vi "RunMe.vi"() -> ()   [LabVIEW 2011]
uses:
  Documenti/Globals.vi
  <vilib>/gmath/NI_Gmath.lvlib
panel:
  in  "Sensor side":enum16{"Right", "Left"}(ring)
  out "Position":dbl(knob) max=500.0 scale=0.0..360.0
  out "home?":bool=TRUE
  in  "Motor on":bool
  out "Measurement OK":bool
  in  "stop":bool
  in  "Tab Control":enum32{"Connect", "Acquire", "Analyze"}(tab)
  in  "Sphere tolerance (mm)":dbl=0.5
  in  "Sphere nominal diameter (mm)":dbl=12.5
  in  "VISA resource name":refnum<visa-resource-name>
  out "pulses":u32
  out "Progress Bar":u32(slide) max=500 scale=-1.0..500.0
  in  "Record Button":bool
  out "data":enum16{"Right", "Left"}(ring)
  out "Current measurement":cluster{dbl[], dbl[]}(graph)
  out "Previus measurements":cluster{dbl[], "best nonlinear fit":dbl[]}[](graph)
  in  "index (page)":i32=1 min=-1 step=1
  out "Residuals":cluster{dbl[], dbl[]}(graph)
  in  "model description":T1={"model"="r+n*sin(x/360*2*3.141593+f)", "Parameters"=["r", "n", "f"], "x"="x"}
  in  "initial parameters":dbl[](array[numeric])=[1.0, 1.0, 1.0]
  out "best fit parameters":dbl[](array[numeric])
  in  "Clear":bool
  out "size(s)":i32
  out "Right":cluster{dbl[], dbl[]}(graph)
  in  "Left measurements":u32(slide) step=1 scale=0.0..9.0
  in  "Right measurements":u32(slide) step=1 scale=0.0..1.0
  out "Left":cluster{dbl[], dbl[]}(graph)
  # "This panel is not complete!"
  # "This panel is not complete!"
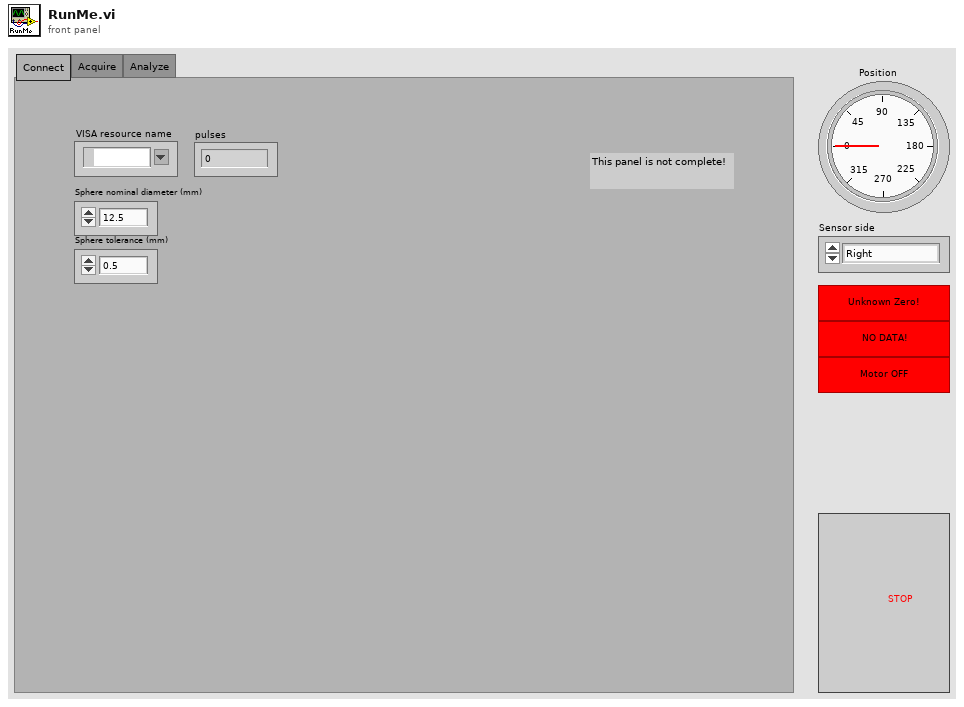
[diagram p1: front panel]
types:
  T1 = cluster{"model":string, "Parameters":string[], "x":string}
  T2 = enum32{"Page Enabled", "Page Disabled", "Page Disabled & Grayed"}
  T3 = enum8{"Enabled", "Disabled", "Disabled and Grayed Out"}
  T4 = cluster{"velocity":dbl, "position":u32, "home?":bool, "reset?":bool, "angle":dbl, "new?":bool}
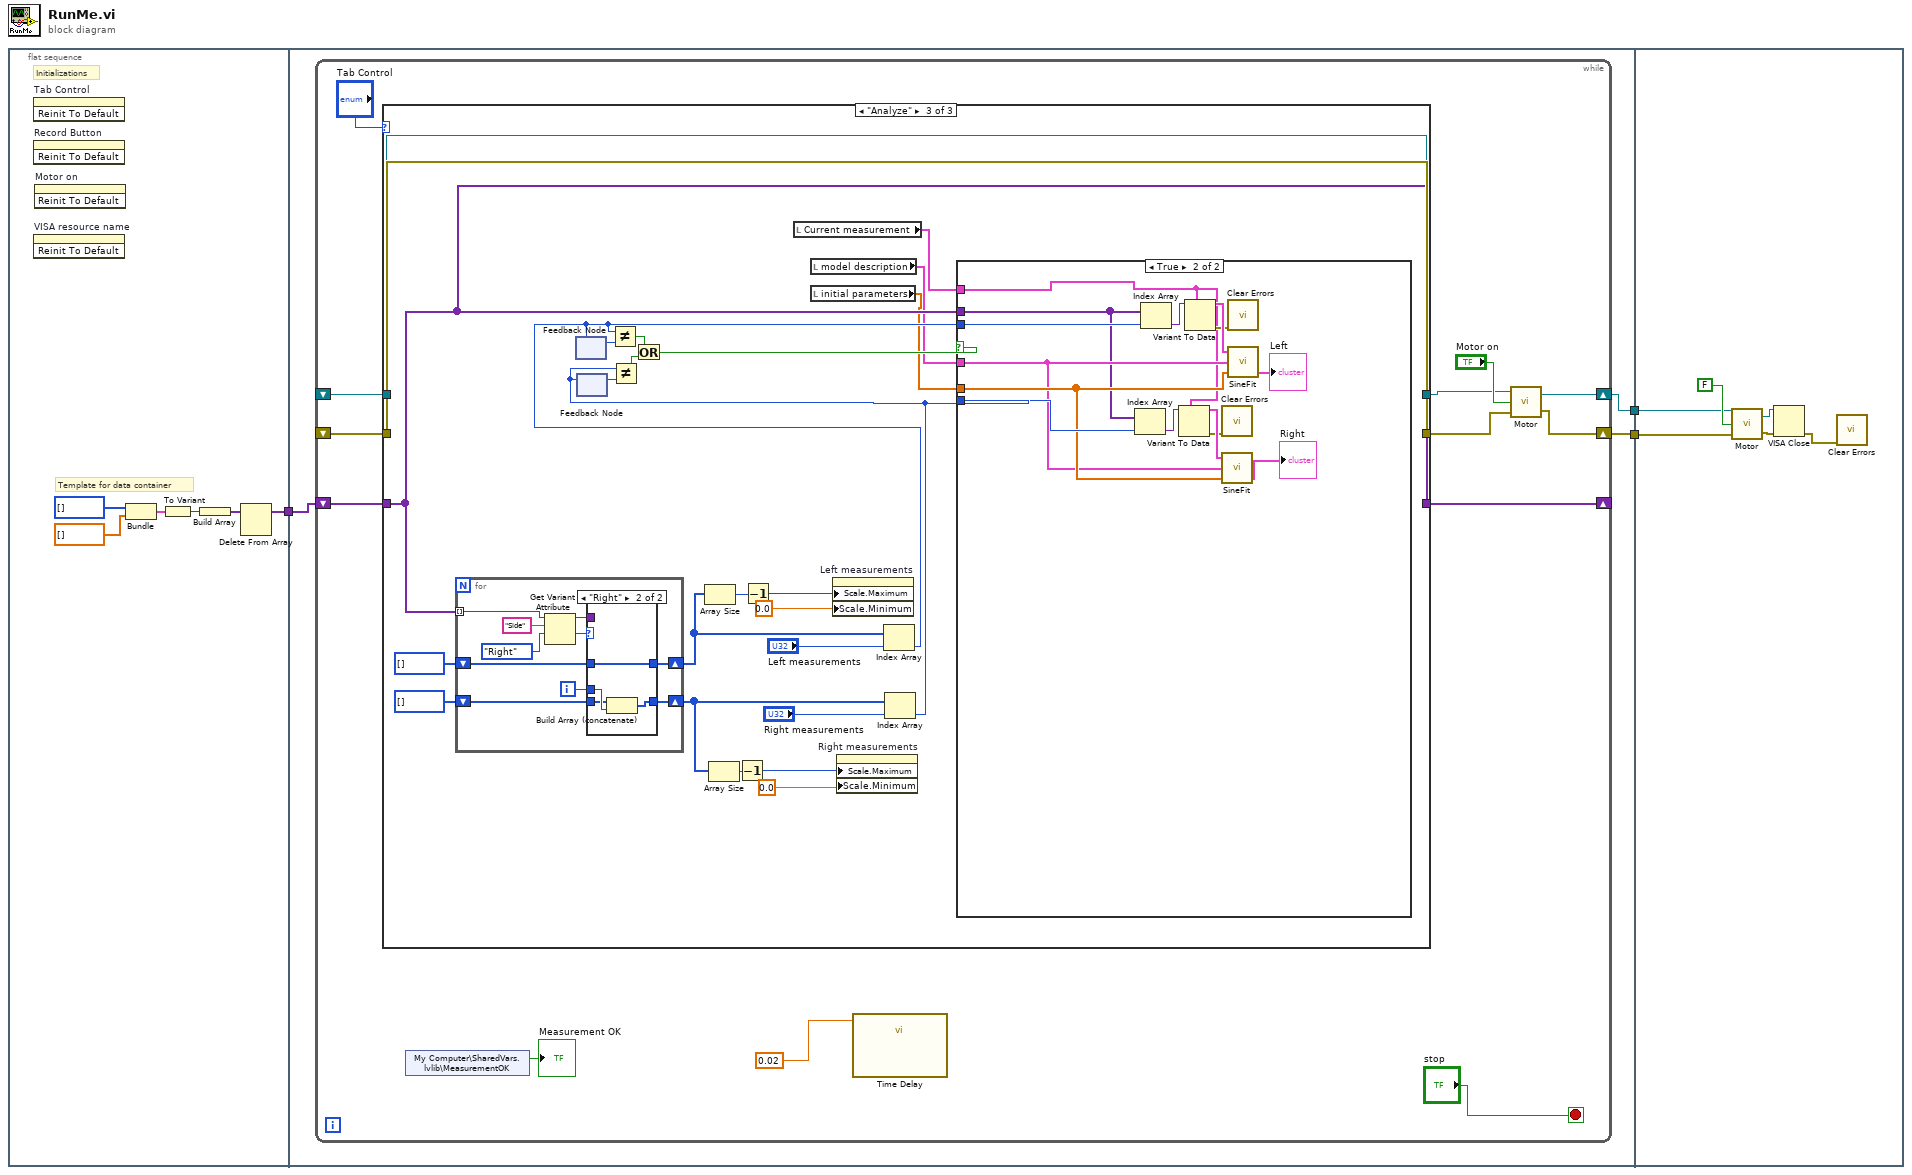
[diagram p0: block diagram]
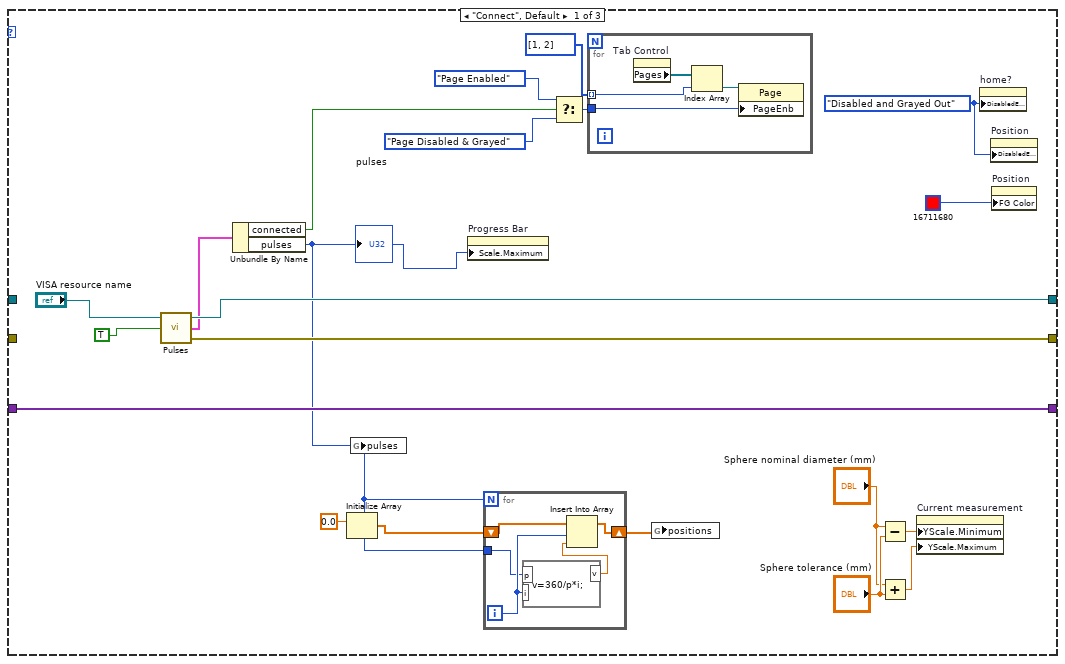
[diagram p2: hidden frame]
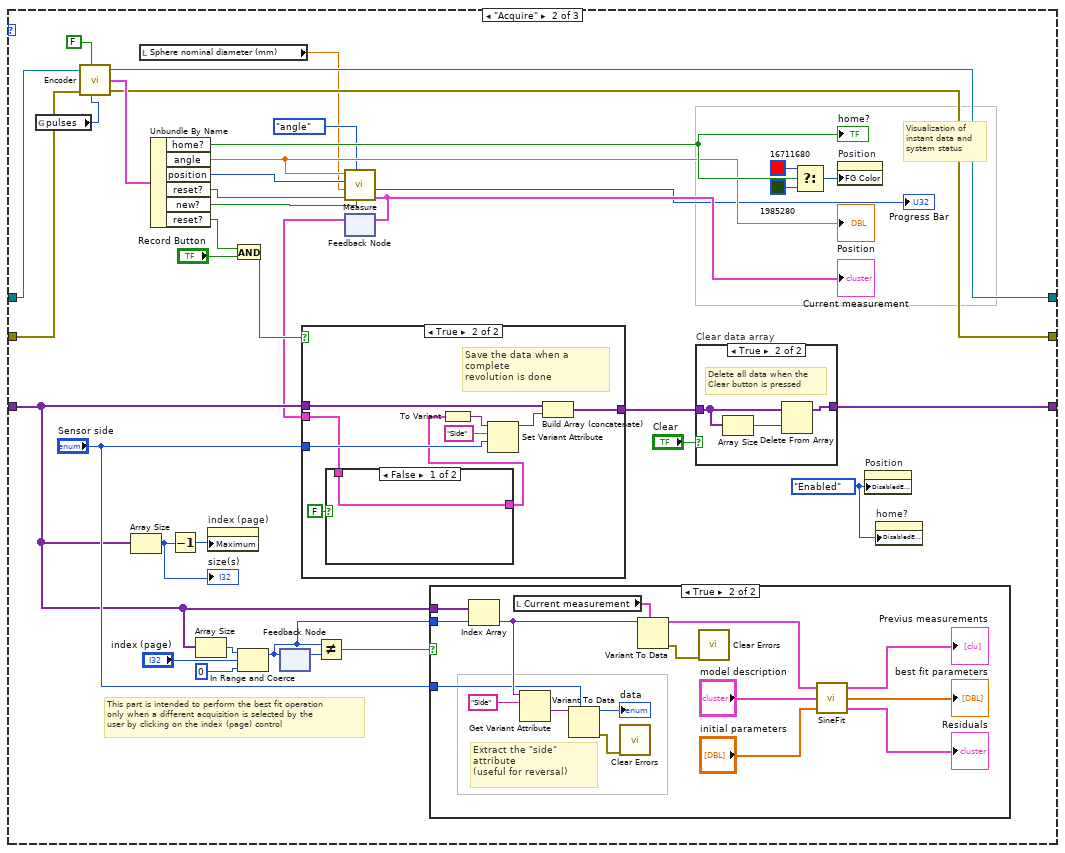
[diagram p3: hidden frame]
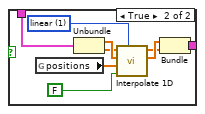
[diagram p7: hidden frame]
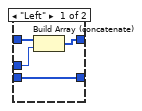
[diagram p9: hidden frame]
diagram:
  n1 = flat-sequence {
    tunnel: [w6] -> w3
    tunnel: w3 -> [w12]
    tunnel: [w11] -> w2
    tunnel: [w10] -> w1
    tunnel: w2 -> [w193]
    tunnel: w1 -> [w192]
    frame #0 {
      # "Initializations"
      # "Template for data container"
      n2 = invoke on="Tab Control" class="TabCtl (strict)" method="Reinit To Default"() -> ()  [unwired: 3 in, 3 out]
      n3 = invoke on="Record Button" class="Bool (strict)" method="Reinit To Default"() -> ()  [unwired: 3 in, 3 out]
      n4 = invoke on="VISA resource name" class="VISAName" method="Reinit To Default"() -> ()  [unwired: 3 in, 3 out]
      n5 = invoke on="Motor on" class="Bool (strict)" method="Reinit To Default"() -> ()  [unwired: 3 in, 3 out]
      n6 = Bundle(u32[] [], dbl[] []) -> (w7:cluster{u32[], dbl[]})  [unwired: 1 in]
      n7 = To Variant(anything=w7) -> (Variant=w8:variant)
      n8 = Build Array(w8) -> (w9:variant[])
      n9 = Delete From Array(array=w9) -> (array with subset deleted=w6:variant[])  [unwired: 2 in, 1 out]
    }
    frame #1 {
      n10 = while {
        shift-right: [w13] -> w10
        shift-left: _ -> [w21]
        shift-right: [w15] -> w11
        shift-left: _ -> [w22]
        shift-right: [w18] -> _
        shift-left: w12 -> [w19]
        stop <- "stop" stop-if-true
        n11 = case shown="\"Analyze\"" "Tab Control" {
          tunnel: [w46 w64 w156] -> w16
          tunnel: [w45 w63 w157] -> w14
          tunnel: w22 -> [_ w87 w156]
          tunnel: w21 -> [_ w86 w157]
          tunnel: w19 -> [w44 w75 w149]
          tunnel: [w44 w85 w149] -> w18
          frame "Connect", Default {
            w35 = T3."Disabled and Grayed Out" ("Disabled")
            n12 = call "Pulses.vi"("try connection?"=TRUE, "VISA resource name in"="VISA resource name") -> ("error out"=w45:errorcluster, "connection result"=w34:cluster{"pulses":i32, "connected":bool}, "VISA resource name out"=w46:refnum<visa-resource-name>)  [unwired: 1 in]
            n13 = Unbundle By Name(w34) -> ("connected"=w31:bool, "pulses"=w26:i32)
            "pulses" <- w26
            n14 = Initialize Array(0.0 ("element")) -> (w28:dbl[])  [unwired: 1 in]
            n15 = global write "Globals.vi" "pulses"(w26) -> ()
            n16 = property on="Progress Bar" class="Slide (strict)"("Scale.Maximum"=w26) -> ()  [unwired: 2 in, 2 out]
            n17 = for {
              N: w26 -> [_]
              tunnel: w26 -> [w47]
              shift-right: [w49] -> w27
              shift-left: w28 -> [w51]
              i -> [w48]
              n18 = formula code="v=360/p*i;"("i"=w48, "p"=w47) -> ("v"=w50:dbl)
              n19 = Insert Into Array(array=w51, index=w48, new element=w50) -> (w49:dbl[])
            }
            n20 = Select(t=T2."Page Enabled" ("Page Enabled State"), s=w31, f=T2."Page Disabled & Grayed" ("Page Enabled State")) -> (s? t:f=w41:T2)
            n21 = for {
              tunnel: w41 -> [w53]
              tunnel: i32[] [1, 2] -> [w52] mode=indexing
              n22 = property on="Tab Control" class="TabCtl (strict)"() -> ("Pages"=w55:refnum<vi>[])  [unwired: 2 in, 2 out]
              n23 = Index Array(array=w55, index=w52) -> (element=w54:refnum<vi>)
              n24 = property class="Page"(reference=w54, "PageEnb"=w53) -> ()  [unwired: 1 in, 2 out]
            }
            n25 = global write "Globals.vi" "positions"(w27) -> ()
            n26 = Subtract(x="Sphere nominal diameter (mm)", y="Sphere tolerance (mm)") -> (x-y=w38:dbl)
            n27 = Add(x="Sphere nominal diameter (mm)", y="Sphere tolerance (mm)") -> (x+y=w39:dbl)
            n28 = property on="Current measurement" class="XYGraph (strict)"("YScale.Minimum"=w38, "YScale.Maximum"=w39) -> ()  [unwired: 2 in, 2 out]
            n29 = property on="home?" class="Bool (strict)"("DisabledEnum"=w35) -> ()  [unwired: 2 in, 2 out]
            n30 = property on="Position" class="Knob (strict)"("DisabledEnum"=w35) -> ()  [unwired: 2 in, 2 out]
            n31 = property on="Position" class="Knob (strict)"("FG Color"=u32 16711680) -> ()  [unwired: 2 in, 2 out]
          }
          frame "Acquire" {
            w62 = T3."Enabled" ("Disabled")
            # "This part is intended to perform the best fit operation\nonly when a different acquisition is selected by the \nuser by clicking on the index (page) control"
            # "Visualization of\ninstant data and\nsystem status"
            n32 = global read "Globals.vi" "pulses"() -> (w56:u32)
            n33 = call "Encoder.vi"("Serial Port in"=w87, "simulate?"=FALSE, "error in"=w86, "pulses"=w56) -> ("Serial Port out"=w64:refnum<visa-resource-name>, "status"=w91:T4, "error out"=w63:errorcluster)  [unwired: 1 in]
            n34 = Array Size(array=w75) -> (size(s)=w74:i32)
            "size(s)" <- w74
            n35 = local read "Sphere nominal diameter (mm)"() -> (w57:dbl)
            n36 = Unbundle By Name(w91) -> ("home?"=w69:bool, "angle"=w67:dbl, "position"=w68:u32, "reset?"=w58:bool, "new?"=w59:bool, "reset?"=w71:bool)
            "home?" <- w69
            "Position" <- w67
            n37 = Decrement(x=w74) -> (x-1=w73:u32)
            n38 = Array Size(array=w75) -> (size(s)=w83:i32)
            n39 = property on="index (page)" class="DigNum (strict)"("Maximum"=w73) -> ()  [unwired: 2 in, 2 out]
            n40 = And(x=w71, y="Record Button") -> (x .and. y?=w70:bool)
            n41 = In Range and Coerce(upper limit=w83, x="index (page)", lower limit=0 ("y")) -> (coerced(x)=w81:i32)  [unwired: 1 out]
            n42 = feedback #1() -> (w88:i32)  [unwired: 1 in]
            n43 = feedback-in #1(w81) -> ()
            n44 = Not Equal?(x=w81, y=w88) -> (x != y?=w82:bool)
            n45 = call "Measure.vi"("new data?"=w59, "position or angle"=enum16{"position", "angle"}."angle", "reset?"=w58, "nominal radius"=w57, "position"=w68, "angle"=w67) -> ("data"=w61:cluster{dbl[], dbl[]}, "count"=→"Progress Bar":u32)  [unwired: 2 out]
            "Current measurement" <- w61
            n46 = feedback-in #2(w61) -> ()
            n47 = feedback #2() -> (w65:cluster{dbl[], dbl[]})  [unwired: 1 in]
            n48 = case shown="True" w70 {
              tunnel: [w113 w121] -> w90
              tunnel: w75 -> [w113 w122]
              tunnel: w65 -> [_ w116]
              tunnel: "Sensor side" -> [_ w117]
              frame False {
              }
              frame True {
                # "Save the data when a complete \nrevolution is done"
                n49 = case shown="False" FALSE {
                  tunnel: w116 -> [w123 w132]
                  tunnel: [w123 w131] -> w115
                  frame False {
                  }
                  frame True {
                    w124 = 1 items=["nearest", "linear", "spline", "cubic Hermite", "Lagrange"] ("method")
                    n50 = global read "Globals.vi" "positions"() -> (w130:dbl[])
                    n51 = Unbundle(w132) -> (w129:dbl[], w128:dbl[])
                    n52 = call <vilib>:"Interpolate 1D.vi"("method"=w124, "X is monotonic"=FALSE, "xi"=w130, "X"=w129, "Y"=w128) -> ("xi used"=w127:dbl[], "yi"=w126:dbl[])  [unwired: 4 in, 1 out]
                    n53 = Bundle("xi used"=w127, "yi"=w126) -> (w131:cluster{"xi used":dbl[], "yi":dbl[]})  [unwired: 1 in]
                  }
                }
                n54 = To Variant(anything=w115) -> (Variant=w120:variant)
                n55 = Set Variant Attribute(Variant=w120, name="Side", value=w117) -> (Variant out=w118:variant)  [unwired: 1 in, 2 out]
                n56 = Build Array (concatenate)(w122, w118) -> (w121:variant[])
              }
            }
            n57 = case shown="True" w82 {
              tunnel: w75 -> [_ w108]
              tunnel: w81 -> [_ w104]
              tunnel: "Sensor side" -> [_ w96]
              frame False {
                # "If the acquisition set is unchanged, does nothing"
              }
              frame True {
                # "Extract the \"side\" attribute\n(useful for reversal)"
                n58 = Index Array(array=w108, index=w104) -> (element=w99:variant)
                n59 = local read "Current measurement"() -> (w93:cluster{dbl[], dbl[]})
                n60 = Get Variant Attribute(Variant=w99, name="Side") -> (value=w97:variant)  [unwired: 2 in, 3 out]
                n61 = Variant To Data(type=w96, Variant=w97) -> (data=→"data":enum16{"Right", "Left"}, error out=w94:errorcluster)  [unwired: 1 in]
                n62 = call <vilib>:"Clear Errors.vi"("error in (no error)"=w94) -> ()  [unwired: 6 in, 1 out]
                n63 = Variant To Data(type=w93, Variant=w99) -> (data=w103:cluster{dbl[], dbl[]}, error out=w100:errorcluster)  [unwired: 1 in]
                n64 = call <vilib>:"Clear Errors.vi"("error in (no error)"=w100) -> ()  [unwired: 6 in, 1 out]
                n65 = call "SineFit.vi"("initial parameters"="initial parameters", "model description"="model description", "data template"=w103) -> ("residuals"=→"Residuals":cluster{dbl[], dbl[]}, "best fit parameters"=→"best fit parameters":dbl[], "chart and fit"=→"Previus measurements":cluster{dbl[], "best nonlinear fit":dbl[]}[])
              }
            }
            n66 = case "Clear data array" shown="True" "Clear" {
              tunnel: w90 -> [w109 w111]
              tunnel: [w109 w110] -> w85
              frame False {
              }
              frame True {
                # "Delete all data when the\nClear button is pressed"
                n67 = Array Size(array=w111) -> (size(s)=w112:i32)
                n68 = Delete From Array(array=w111, length=w112) -> (array with subset deleted=w110:variant[])  [unwired: 1 in, 1 out]
              }
            }
            n69 = Select(t=u32 16711680, s=w69, f=u32 1985280) -> (s? t:f=w76:u32)
            n70 = property on="Position" class="Knob (strict)"("FG Color"=w76) -> ()  [unwired: 2 in, 2 out]
            n71 = property on="Position" class="Knob (strict)"("DisabledEnum"=w62) -> ()  [unwired: 2 in, 2 out]
            n72 = property on="home?" class="Bool (strict)"("DisabledEnum"=w62) -> ()  [unwired: 2 in, 2 out]
          }
          frame "Analyze" {
            n73 = for {
              tunnel: w149 -> [w181] mode=indexing
              shift-right: [w173] -> w143
              shift-left: i32[] [] -> [w175]
              shift-right: [w172] -> w147
              shift-left: i32[] [] -> [w174]
              i -> [w176]
              n74 = Get Variant Attribute(Variant=w181, name="Side", default value (empty Variant)=enum16{"Right", "Left"}."Right" ("Sensor side")) -> (duplicate Variant=w177:variant, value=w179:enum16{"Right", "Left"})  [unwired: 1 in, 2 out]
              n75 = case shown="\"Right\"" w179 {
                tunnel: w177 -> [_ _]
                tunnel: w176 -> [w185 w189]
                tunnel: [w182 w188] -> w173
                tunnel: [w184 w187] -> w172
                tunnel: w175 -> [w182 w186]
                tunnel: w174 -> [w183 w187]
                frame "Left" {
                  n76 = Build Array (concatenate)(w183, w185) -> (w184:i32[])
                }
                frame "Right" {
                  n77 = Build Array (concatenate)(w186, w189) -> (w188:i32[])
                }
              }
            }
            n78 = feedback #3() -> (w146:i32)  [unwired: 1 in]
            n79 = feedback #4() -> (w142:i32)  [unwired: 1 in]
            n80 = Array Size(array=w147) -> (size(s)=w153:i32)
            n81 = Array Size(array=w143) -> (size(s)=w152:i32)
            n82 = Decrement(x=w152) -> (x-1=w133:i32)
            n83 = Decrement(x=w153) -> (x-1=w134:i32)
            n84 = local read "Current measurement"() -> (w137:cluster{dbl[], dbl[]})
            n85 = local read "model description"() -> (w136:T1)
            n86 = local read "initial parameters"() -> (w135:dbl[])
            n87 = property on="Left measurements" class="Slide (strict)"("Scale.Maximum"=w134, "Scale.Minimum"=0.0 ("Scale.Range:Minimum")) -> ()  [unwired: 2 in, 2 out]
            n88 = property on="Right measurements" class="Slide (strict)"("Scale.Maximum"=w133, "Scale.Minimum"=0.0 ("Scale.Range:Minimum")) -> ()  [unwired: 2 in, 2 out]
            n89 = Index Array(array=w147, index="Left measurements") -> (element=w145:i32)
            n90 = feedback-in #3(w145) -> ()
            n91 = Not Equal?(x=w145, y=w146) -> (x != y?=w140:bool)
            n92 = Index Array(array=w143, index="Right measurements") -> (element=w138:i32)
            n93 = feedback-in #4(w138) -> ()
            n94 = Not Equal?(x=w138, y=w142) -> (x != y?=w141:bool)
            n95 = Or(x=w140, y=w141) -> (x .or. y?=w139:bool)
            n96 = case shown="True" w139 {
              tunnel: w149 -> [_ w160]
              tunnel: w145 -> [_ w168]
              tunnel: w138 -> [_ w163]
              tunnel: w137 -> [_ w159]
              tunnel: w136 -> [_ w161]
              tunnel: w135 -> [_ w162]
              frame False {
              }
              frame True {
                n97 = Index Array(array=w160, index=w163) -> (element=w164:variant)
                n98 = Index Array(array=w160, index=w168) -> (element=w167:variant)
                n99 = Variant To Data(type=w159, Variant=w164) -> (data=w166:cluster{dbl[], dbl[]}, error out=w165:errorcluster)  [unwired: 1 in]
                n100 = Variant To Data(type=w159, Variant=w167) -> (data=w171:cluster{dbl[], dbl[]}, error out=w169:errorcluster)  [unwired: 1 in]
                n101 = call <vilib>:"Clear Errors.vi"("error in (no error)"=w165) -> ()  [unwired: 6 in, 1 out]
                n102 = call "SineFit.vi"("initial parameters"=w162, "model description"=w161, "data template"=w166) -> ("residuals"=→"Right":cluster{dbl[], dbl[]})  [unwired: 2 out]
                n103 = call <vilib>:"Clear Errors.vi"("error in (no error)"=w169) -> ()  [unwired: 6 in, 1 out]
                n104 = call "SineFit.vi"("initial parameters"=w162, "model description"=w161, "data template"=w171) -> ("residuals"=→"Left":cluster{dbl[], dbl[]})  [unwired: 2 out]
              }
            }
          }
        }
        n105 = shared-variable "My Computer\\SharedVars.lvlib\\MeasurementOK"() -> (→"Measurement OK":bool)  [unwired: 1 in, 1 out]
        n106 = call "Time Delay"("Delay Time (s)"=0.02) -> ()  [unwired: 10 in, 1 out]
        n107 = call "Motor.vi"("error in"=w14, "Motor on?"="Motor on", "Serial Port in"=w16) -> ("error out"=w13:errorcluster, "Serial Port out"=w15:refnum<visa-resource-name>)
      }
    }
    frame #2 {
      n108 = call "Motor.vi"("error in"=w192, "Motor on?"=FALSE ("Motor on 2"), "Serial Port in"=w193) -> ("error out"=w194:errorcluster, "Serial Port out"=w191:refnum<visa-resource-name>)
      n109 = VISA Close(VISA resource name=w191, error in (no error)=w194) -> (error out=w190:errorcluster)
      n110 = call <vilib>:"Clear Errors.vi"("error in (no error)"=w190) -> ()  [unwired: 6 in, 1 out]
    }
  }
